vi "Auton Drive Gyro & Encoder.vi"(4 "Left Gains":T1={"proportional gain (Kc)"=0.25, "integral time (Ti, min)"=0.0, "derivative time (Td, min)"=0.0} {"derivative time (Td, min)" format="%.3f"; "integral time (Ti, min)" format="%.3f"; "proportional gain (Kc)" format="%.3f"}, 5 "Right Gains":T1={"proportional gain (Kc)"=0.25, "integral time (Ti, min)"=0.0, "derivative time (Td, min)"=0.0} {"derivative time (Td, min)" format="%.3f"; "integral time (Ti, min)" format="%.3f"; "proportional gain (Kc)" format="%.3f"}, 6 "Left Range":cluster{"output high":dbl, "output low":dbl}={"output high"=0.6, "output low"=-0.6} {"output low" format="%.2f"; "output high" format="%.2f"}, 7 "Right Range":cluster{"output high":dbl, "output low":dbl}={"output high"=0.6, "output low"=-0.6} {"output low" format="%.2f"; "output high" format="%.2f"}, 8 "Angle Setpoint":dbl=90.0, 10 "Right Set Point":dbl, 11 "Left Set Point":dbl=-200.0) -> (3 "At Destination?":bool=TRUE)   [LabVIEW 2014]
uses:
  <vilib>/Rock Robotics/WPI/RobotDrive/WPI_RobotDriveGetSetRefNum.vi
  <vilib>/addons/control/pid/pid.llb/PID (DBL).vi
  <vilib>/Rock Robotics/Network Tables/SD Write Number.vi
  <vilib>/Rock Robotics/WPI/RobotDrive/WPI_RobotDriveArcadeDrive_ButtonSpin.vi
  <vilib>/addons/control/pid/NI_PID_pid.lvlib
panel:
  out "Array 2":bool[](array[boolean])
  out "Array":bool[](array[boolean])
  out "in range gyro?":bool
  out "in range encoder?":bool
  in  "Gyro Destination Range":dbl=1.0
  out "Y Value Forward/Rev":dbl=0.6 format="%.2f"
  in  "Gyro Gains":T1={"proportional gain (Kc)"=0.07, "integral time (Ti, min)"=0.0, "derivative time (Td, min)"=0.0} {"derivative time (Td, min)" format="%.3f"; "integral time (Ti, min)" format="%.3f"; "proportional gain (Kc)" format="%.3f"}
  in  "Gyro Range":cluster{"output high":dbl, "output low":dbl}={"output high"=0.5, "output low"=-0.5} {"output low" format="%.2f"; "output high" format="%.2f"}
  out "Gyro Reading":dbl(knob)=95.22019510563 scale=-180.0..180.0
  out "X Value Left/Right Correction":dbl=-0.36541365739409987 format="%.2f"
  in  "Encoder Destination Range":dbl=2.0
  in  "Gain (VoltsPerDegree/Second)":dbl=0.0066
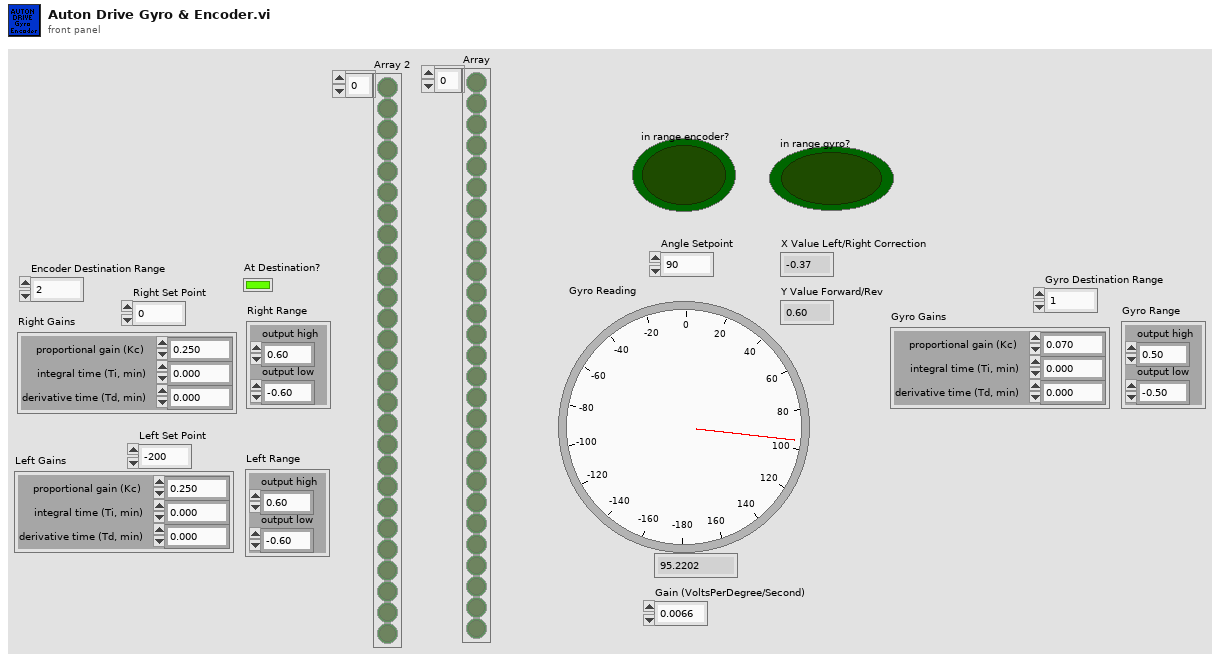
[diagram p1: front panel]
types:
  T1 = cluster{"proportional gain (Kc)":dbl, "integral time (Ti, min)":dbl, "derivative time (Td, min)":dbl}
  T2 = typedef "WPI_GyroDevRef.ctl" = cluster{"DevStatus":errorcluster, "Analog Module":T3, "Analog Channel":T4, "Offset":dbl, "Gain (VoltsPerDegree/Second)":dbl}
  T3 = typedef "FPGA_TypedefAnalogModule.ctl" = enum16{"Controller 1"}
  T4 = typedef "FPGA_AIChannel.ctl" = enum8{"AI 0", "AI 1", "AI 2", "AI 3", "AI MXP 0", "AI MXP 1", "AI MXP 2", "AI MXP 3", "Invalid"}
  T5 = typedef "WPI_EncoderDevRef.ctl" = cluster{"DevStatus":errorcluster, "EncoderIndex":T6, "CounterIndex":T7, "DistancePerCount":dbl, "Decoding Type":T8}
  T6 = typedef "FPGA_EncoderIdx.ctl" = enum8{"Enc 0", "Enc 1", "Enc 2", "Enc 3", "Enc 4", "Enc 5", "Enc 6", "Enc 7", "Invalid"}
  T7 = typedef "FPGA_CounterCtrSystemIndex.ctl" = enum8{"Ctr 0", "Ctr 1", "Ctr 2", "Ctr 3", "Ctr 4", "Ctr 5", "Ctr 6", "Ctr 7", "Invalid"}
  T8 = typedef "WPI_EncoderType.ctl" = enum16{"1x", "2x", "4x"}
  T9 = typedef "WPI_RobotDriveDevRef.ctl" = cluster{"DevStatus":errorcluster, "Motors[]":T10[], "Square Inputs":bool, "Max Output":dbl}
  T10 = typedef "WPI_MotorControlDeviceRef.ctl" = cluster{"DeviceStatus":errorcluster, "Type":T11, "PWM":cluster{"Controller":T12, "PWM Channel":T13, "DeadBand":T14}, "CAN":cluster{"Device Number":u8, "Control Mode":T15, "Semaphore":T16, "Max Vout":dbl, "TalonSRX Control Mode":T17}, "Invert":bool, "TransformRef":T18, "InvTransformRef":T18}
  T11 = typedef "WPI_MotorControlType.ctl" = enum16{"PWM", "CAN", "CANTalonSRX"}
  T12 = typedef "FPGA_TypedefDigitalModule.ctl" = enum16{"Controller 1"}
  T13 = typedef "FPGA_DIOPWMChannel.ctl" = enum8{"PWM 0", "PWM 1", "PWM 2", "PWM 3", "PWM 4", "PWM 5", "PWM 6", "PWM 7", "PWM 8", "PWM 9", "PWM MXP 0", "PWM MXP 1", "PWM MXP 2", "PWM MXP 3", "PWM MXP 4", "PWM MXP 5", "PWM MXP 6", "PWM MXP 7", "PWM MXP 8", "PWM MXP 9", "Invalid"}
  T14 = typedef "WPI_PWMDeadband.ctl" = cluster{"Name":string, "maxPositivePwm":i32, "minPositivePwm":i32, "centerPwm":i32, "maxNegativePwm":i32, "minNegativePwm":i32, "angularRange":u16}
  T15 = typedef "WPI_CANJaguar_ControlMode.ctl" = enum8{"Percent VBus", "Current", "Speed", "Position", "Voltage"}
  T16 = typedef "Semaphore RefNum" = refnum<k1>
  T17 = typedef "WPI_CANTalonSRX_APIControlMode.ctl" = enum8{"Percent VBus", "Speed", "Position", "Slave", "Unchanged / Invalid"}
  T18 = typedef "WPI_PWMTransform_ConPane.ctl" = refnum<vi>
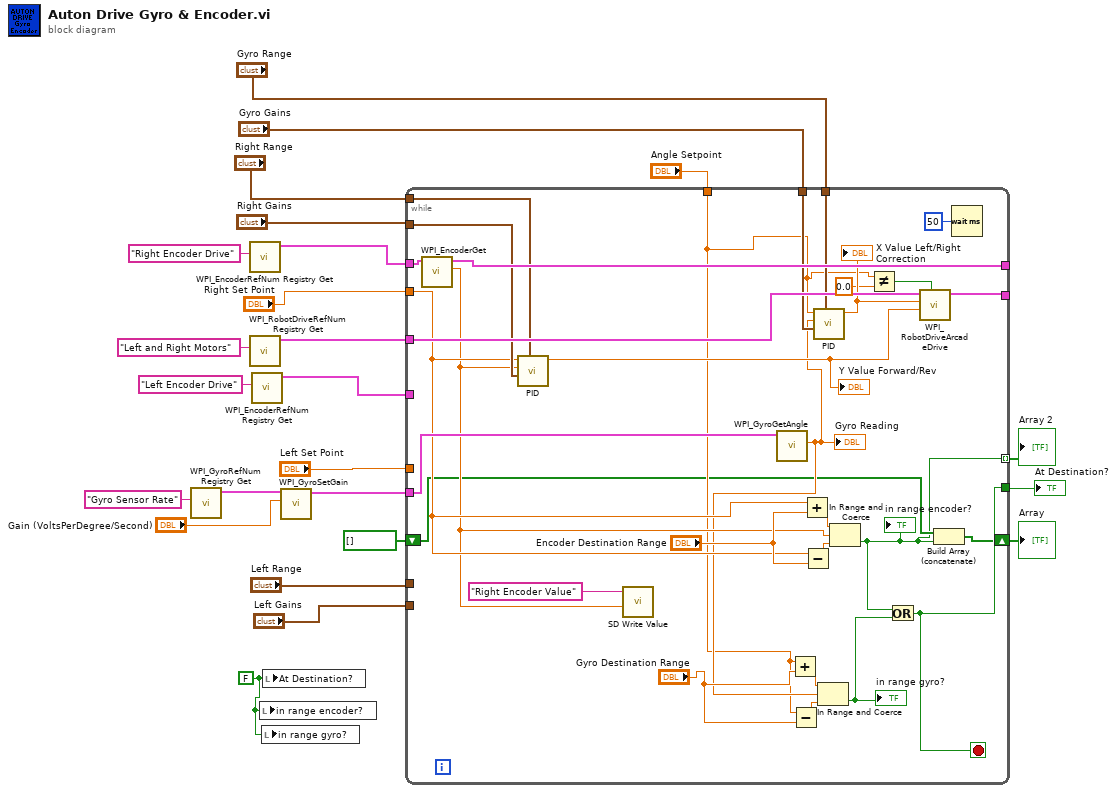
[diagram p0: block diagram]
diagram:
  w5 = FALSE ("At Destination?")
  n1 = call <vilib>:"WPI_GyroRefNum Registry Get.vi"("refnum name"="Gyro Sensor Rate") -> ("GyroDevRef"=w11:T2)  [unwired: 9 in, 1 out]
  n2 = call <vilib>:"WPI_EncoderRefNum Registry Get.vi"("refnum name"="Right Encoder Drive") -> ("EncoderDevRef"=w17:T5)  [unwired: 9 in, 1 out]
  n3 = call <vilib>:"WPI_RobotDriveRefNum Registry Get.vi"("refnum name"="Left and Right Motors") -> ("RobotDriveDevRef"=w21:T9)  [unwired: 9 in, 1 out]
  n4 = call <vilib>:"WPI_EncoderRefNum Registry Get.vi"("refnum name"="Left Encoder Drive") -> ("EncoderDevRef"=w18:T5)  [unwired: 9 in, 1 out]
  n5 = local write "in range encoder?"(w5) -> ()
  n6 = local write "in range gyro?"(w5) -> ()
  n7 = local write "At Destination?"(w5) -> ()
  n8 = call <vilib>:"WPI_GyroSetGain.vi"("Gain (VoltsPerDegree/Second)"="Gain (VoltsPerDegree/Second)", "GyroDevRef"=w11) -> ("GyroDevRef"=w10:T2)  [unwired: 1 in, 8 out]
  n9 = while {
    tunnel: [w53] -> _
    tunnel: [w46] -> _
    tunnel: "Left Gains" -> [_]
    tunnel: "Left Range" -> [_]
    tunnel: w21 -> [w45]
    tunnel: w18 -> [_]
    tunnel: w17 -> [w52]
    tunnel: "Left Set Point" -> [_]
    tunnel: "Right Set Point" -> [w39]
    tunnel: [w30] -> w14
    tunnel: w10 -> [w48]
    tunnel: "Right Range" -> [w41]
    tunnel: "Right Gains" -> [w40]
    tunnel: "Gyro Range" -> [w43]
    tunnel: "Gyro Gains" -> [w42]
    tunnel: "Angle Setpoint" -> [w28]
    shift-right: [w27] -> w2
    shift-left: bool[] [] -> [w26]
    tunnel: [w25] -> w1 mode=indexing
    stop <- w30 stop-if-true
    n10 = call <vilib>:"WPI_EncoderGet.vi"("EncoderDevRef"=w52) -> ("Distance"=w38:dbl, "EncoderDevRef"=w53:T5)  [unwired: 5 in, 4 out]
    n11 = call-poly <vilib>:"PID.vi"("output range"=w41, "PID gains"=w40, "process variable"=w38, "setpoint"=w39) -> ("output"=w37:dbl)  [unwired: 6 in, 1 out]
    "Y Value Forward/Rev" <- w37
    n12 = call-poly <vilib>:"SD Write Value.vi"("Numeric"=w38, "Name"="Right Encoder Value") -> ()  [unwired: 8 in, 2 out]
    n13 = call <vilib>:"WPI_GyroGetAngle.vi"("GyroDevRef"=w48) -> ("Angle"=w31:dbl)  [unwired: 1 in, 9 out]
    "Gyro Reading" <- w31
    n14 = Add(x=w28, y="Gyro Destination Range") -> (x+y=w33:dbl)
    n15 = Subtract(x=w28, y="Gyro Destination Range") -> (x-y=w34:dbl)
    n16 = Add(x=w39, y="Encoder Destination Range") -> (x+y=w51:dbl)
    n17 = Subtract(x=w39, y="Encoder Destination Range") -> (x-y=w50:dbl)
    n18 = call-poly <vilib>:"PID.vi"("output range"=w43, "PID gains"=w42, "process variable"=w31, "setpoint"=w28) -> ("output"=w44:dbl)  [unwired: 6 in, 1 out]
    "X Value Left/Right Correction" <- w44
    n19 = In Range and Coerce(upper limit=w33, x=w31, lower limit=w34) -> (In Range?=w29:bool)  [unwired: 1 out]
    "in range gyro?" <- w29
    n20 = In Range and Coerce(upper limit=w51, x=w38, lower limit=w50) -> (In Range?=w25:bool)  [unwired: 1 out]
    "in range encoder?" <- w25
    n21 = Not Equal?(x=w28, y=0.0) -> (x != y?=w35:bool)
    n22 = Or(x=w25, y=w29) -> (x .or. y?=w30:bool)
    n23 = call-poly <vilib>:"WPI_RobotDriveArcadeDrive.vi"("Spin?"=w35, "Y axis value"=w37, "X axis value"=w44, "RobotDriveDevRef"=w45) -> ("RobotDriveDevRef"=w46:T9)  [unwired: 5 in, 2 out]
    n24 = Build Array (concatenate)(w26, w25) -> (w27:bool[])
    n25 = Wait (ms)(milliseconds to wait=u32 50) -> ()  [unwired: 1 out]
  }
  "At Destination?" <- w14
  "Array" <- w2
  "Array 2" <- w1
